vi "Motion_xbee_1Radar.vi"(0 "VISA resource name":refnum<visa-resource-name>="COM1", 1 "baud rate":u32=9600, 4 "data bits":u16=8 min=5 max=8 step=1, 5 "parity":u16(ring) items=["None", "Odd", "Even", "Mark", "Space"], 7 "stop bits":u16=10, 9 "XON Character":u8=17 format="%.0x", 14 "XOFF Character":u8=19 format="%.0x", 15 "timeout (ms)":u32=10000, 21 "End read on termination character?":bool, 24 "termination char\n(0xA = '\\n' = LF)":u8=10 format="%.0x", 25 "buffer size":u32=4096) -> ()   [LabVIEW 2015]
doc: "The Advanced Serial Read and Write example performs a Serial Port Read, a Serial Port Write, or a combination of these actions while setting some advanced serial features like buffer size, termination characters, and XON/XOFF flow control. The user selects the actions (read or write) on the front panel. If both are selected, the VI will write the data first, read the data and then close the VISA session that is opened to the port. \n\nThe parameters set for the serial port must match the parameters of the connected instrument or device. In this example, the bytes to read parameter specifies the number of bytes that the serial port reads. If there were more bytes at the port than the number specified in bytes to read, those bytes would not be read. Also, if you specify to read more bytes than the number of bytes actually read, you might receive a timeout error message.\n\nINSTRUCTIONS:\n1) Select the serial resource and configuration parameters (baud rate, data bits, parity, stop bits, flow control).\n2) Termination character can be enabled and set. Also, set the required input buffer size prior to running the example.\n3) Select the operations to be performed. \n4) Connect the serial port to your device. If no device is available, perform a loopback test by doing one of the following. Short pins 2 and 3 on a RS-232 cable or short pin 4 to pin 8 and pin 5 to pin 9 on a RS-485/422 cable. \n5) Run the VI to see the data read. (The \"read string\" will match the \"string to write\" if a loopback test was performed.)\n\nThis example exposes several advanced features that you may need for your application. Not all applications need all the features shown in this example. The input buffer size is likely an important setting that you want to control in your application. This example expands upon the flow control option for XON and XOFF, allowing the user to choose those control characters. The timeout parameter has been brought to the front panel so a user can specify the time period the VISA Read will wait for the number of bytes to read before timing out. Also, the user has several controls for the termination character, which is discussed later.\n\nNote that you can press the write and read buttons and change the bytes to read parameters on the fly, while the example is running. However, you must stop the example to change the other configuration parameters after the example has started running, and then run again.\n\nSet the I/O buffer size slightly higher the amount of data you expect to receive. This is very important for applications that don't use flow control, as you may lose characters if the receive buffer overflows.\n\nSetting the timeout period ensures that the operation returns with a timeout error if the operation cannot be performed in the specified time period. \n\nSome devices require a termination character in order to identify the end of command strings. Some devices send a termination character to signify the end of data to be read. \n\nThis example shows how you can end the Read operation once a termination character is detected in the buffer and/or append a termination character at the end of the Write data. To enable the Read to end on a termination character, use the VISA Configure Serial Port or use the VISA Properties Serial End Mode for Reads, Termination Character Enable, and Termination Character. To end the Write with a termination character, use the VISA Properties Serial End Mode for Writes, the Send End Enable, and Termination Character. In this example, the same termination character is used for both the Read and the Write. You can specify two different characters for your application, if desired.\n\nYour application may require specific characters for the XON/XOFF Flow Control. You can specify these characters with the VISA Properties Flow Control XOFF Character and Flow Control XON Character. Note that if the standard XON and XOFF characters are used, then decimal 17 and 19 are unavailable for data values. Remember that using flow control and setting an adequate buffer size allow you to prevent buffer overflows."
uses:
  <vilib>/Analysis/2dsp.llb/Real FFT.vi
  <vilib>/Instr/_visa.llb/VISA Configure Serial Port (Instr).vi
  <vilib>/measure/madcrms.llb/Basic Averaged DC-RMS for 1 Chan.vi
  <vilib>/measure/NI_MAPro.lvlib
  <vilib>/Analysis/NI_AALPro.lvlib
panel:
  in  "Data saving path":path=path "C:/Users/zpeng/OneDrive - Texas Tech University/Desktop"
  in  "Save raw data":bool
  out "Spectrum":waveform(dbl)(graph)
  out "I/Q channels":waveform(dbl)(graph)
  in  "time":timestamp=timestamp(3198752888.296 s since 1904-01-01)
  in  "FFT":i32=800
  in  "flow control":u16(ring) items=["None"=0, "XON/XOFF"=1, "RTS/CTS"=2, "DTR/DSR"=4]
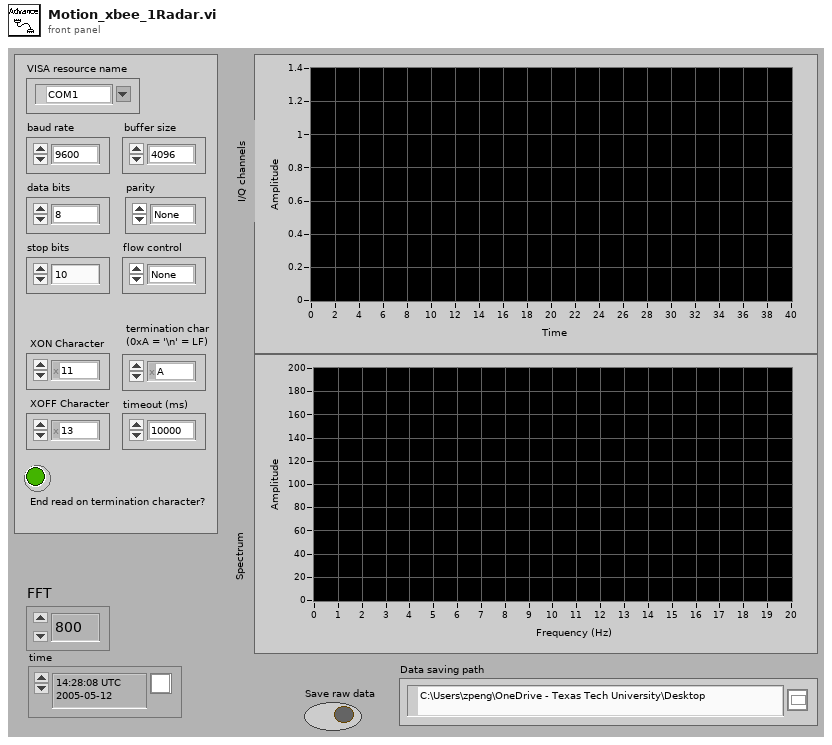
[diagram p1: front panel]
types:
  T1 = enum16{"open", "replace", "create", "open or create", "replace or create", "replace or create with confirmation"}
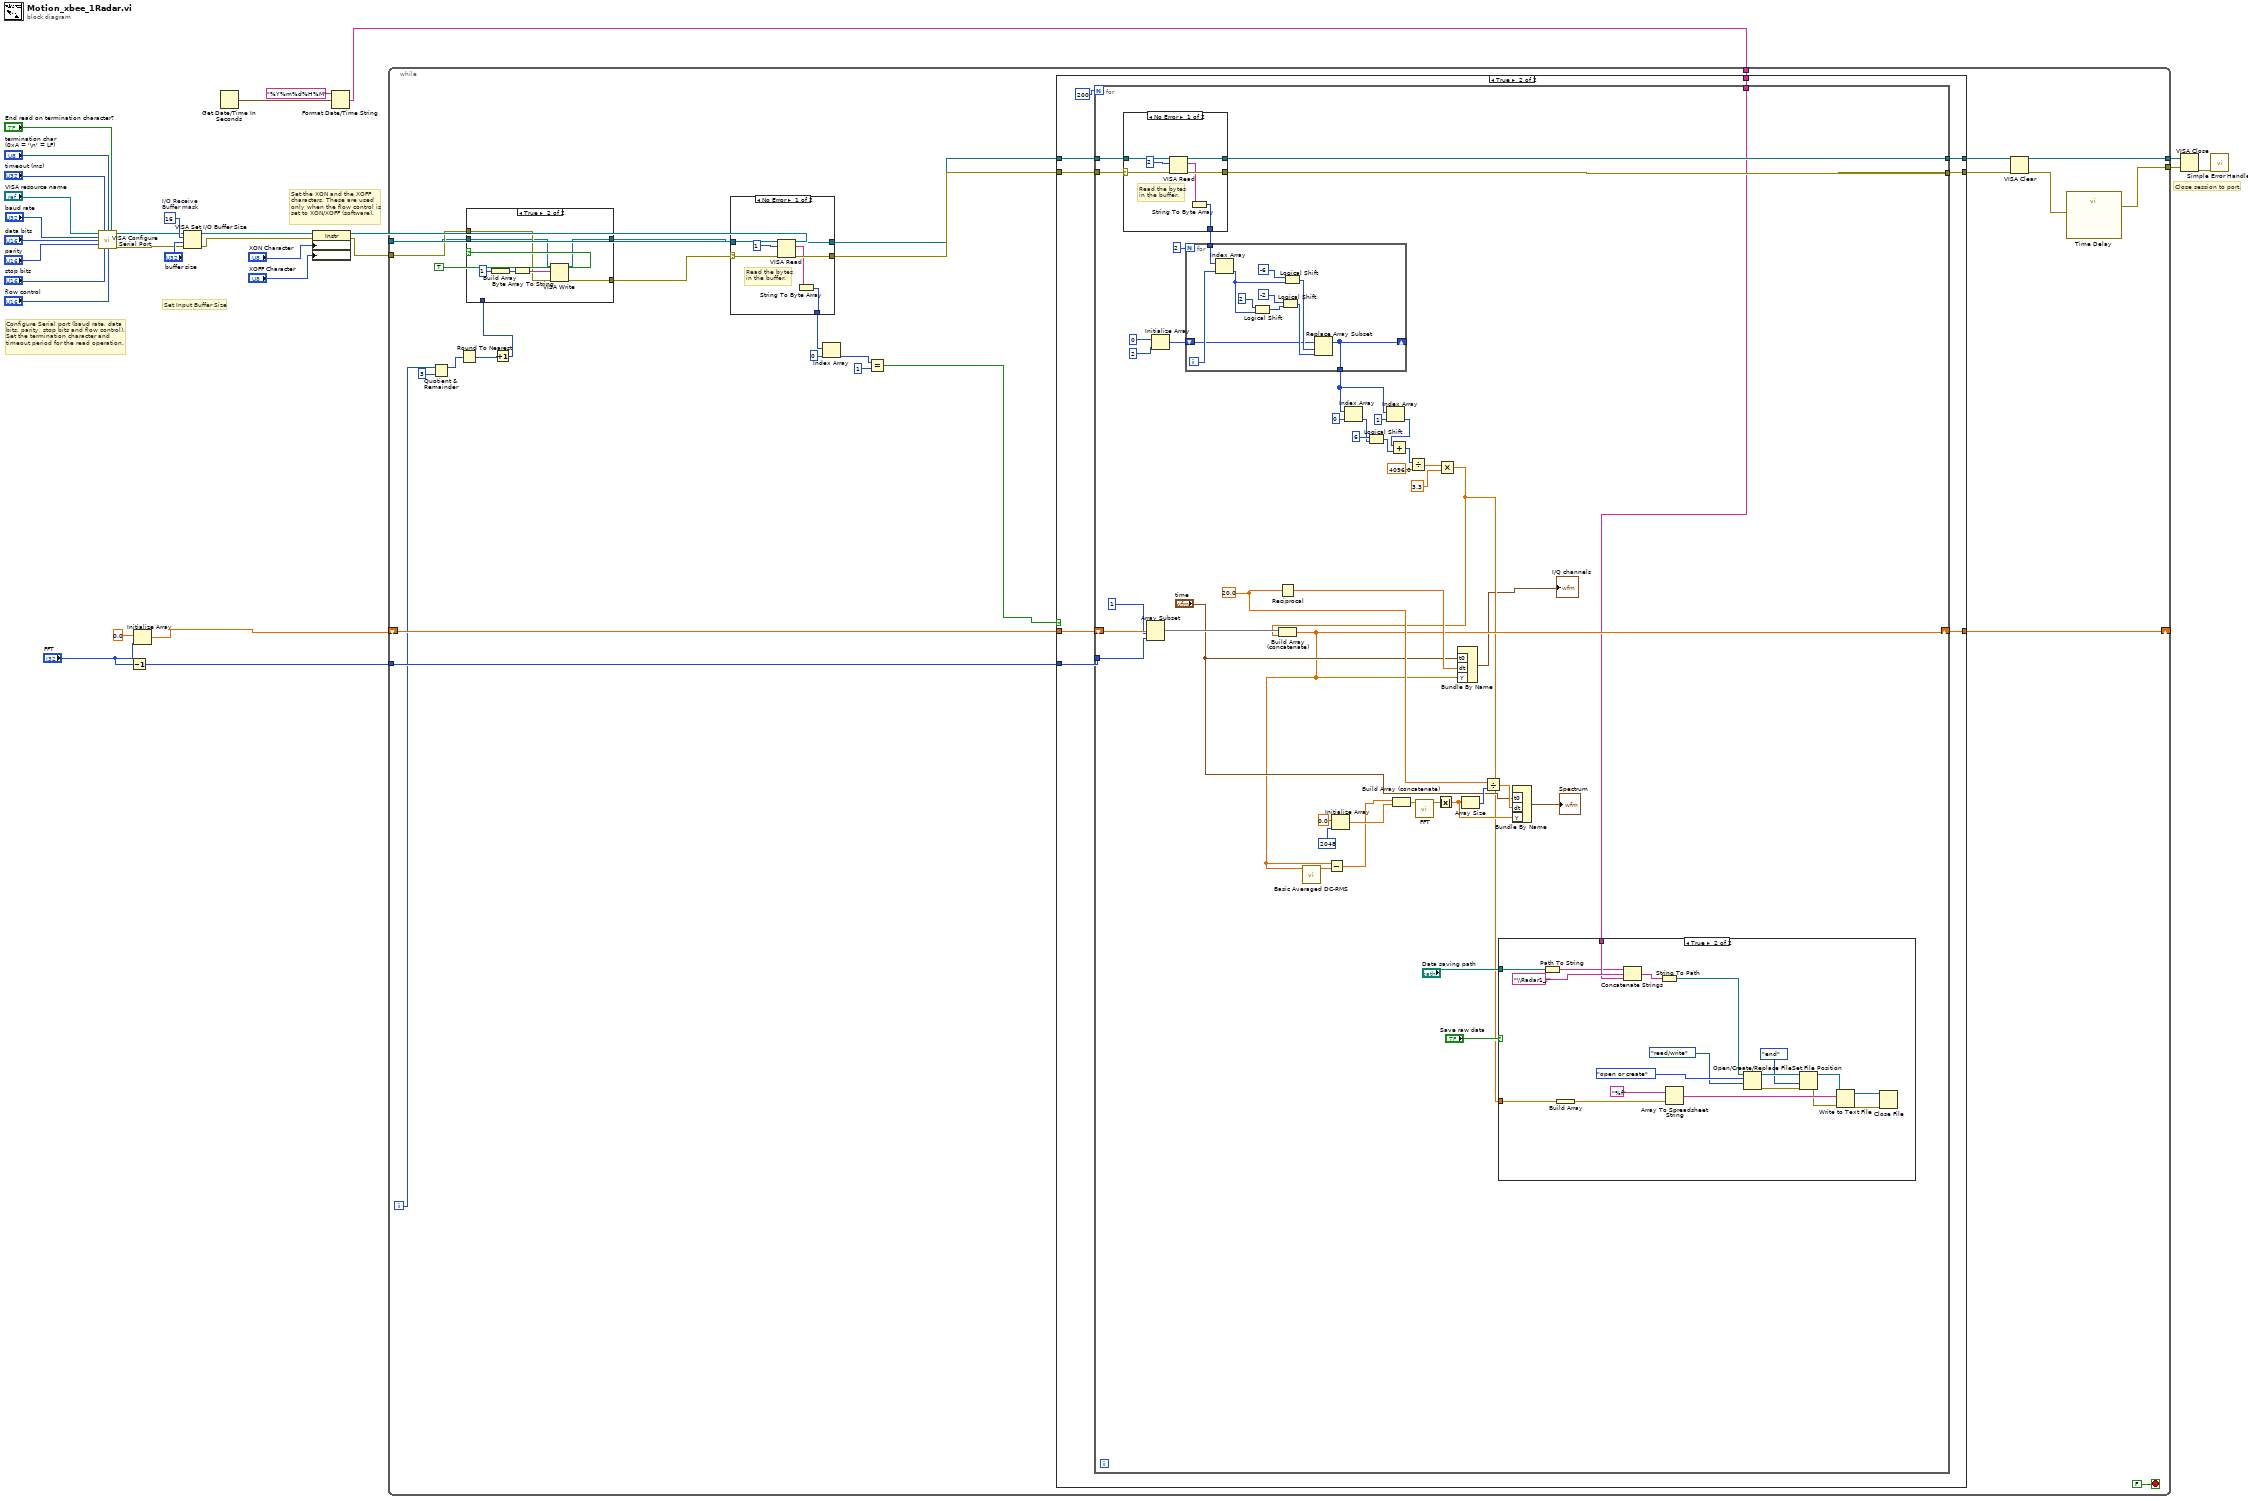
[diagram p0: block diagram]
diagram:
  w22 = u16 16  # I/O Receive Buffer mask
  # "Set the XON and the XOFF\ncharacters. These are used\nonly when the flow control is\nset to XON/XOFF (software)."
  # "Configure Serial port (baud rate, data\nbits, parity, stop bits and flow control).\nSet the termination character and\ntimeout period for the read operation."
  # "Set Input Buffer Size"
  # "Close session to port."
  n1 = call-poly "VISA Configure Serial Port"("VISA resource name"="VISA resource name", "timeout (10sec)"="timeout (ms)", "termination char\n(0xA = '\\n' = LF)"="termination char\n(0xA = '\\n' = LF)", "Enable Termination\nChar (T)"="End read on termination character?", "baud rate (9600)"="baud rate", "data bits (8)"="data bits", "parity (0:none)"="parity", "stop bits (10: 1 bit)"="stop bits", "flow control (0:none)"="flow control") -> ("VISA resource name out"=w8:refnum<visa-resource-name>, "error out"=w7:errorcluster)  [unwired: 1 in, 4 out]
  n2 = Decrement(x="FFT") -> (x-1=w11:i32)
  n3 = Initialize Array(0.0 ("element"), "FFT") -> (w6:dbl[])
  n4 = VISA Set I/O Buffer Size(VISA resource name=w8, mask (16)=w22, size (4096)="buffer size", error in (no error)=w7) -> (VISA resource name out=w18:refnum<visa-resource-name>, error out=w17:errorcluster)
  n5 = Get Date/Time In Seconds() -> (seconds since 1Jan1904=w2:timestamp)
  n6 = property class="Instr"(reference=w18, error in=w17, "Serial Settings:Flow Control XON Character"="XON Character", "Serial Settings:Flow Control XOFF Character"="XOFF Character") -> (reference out=w5:refnum<visa-resource-name>, error out=w4:errorcluster)
  n7 = Format Date/Time String(time format string (%c)="%Y%m%d%H%M", seconds (now)=w2) -> (date/time string=w1:string)  [unwired: 1 in]
  n8 = while {
    tunnel: w11 -> [w56]
    tunnel: w5 -> [w51]
    tunnel: [w45] -> w13
    tunnel: w4 -> [w52]
    tunnel: [w49] -> w12
    shift-right: [w53] -> _
    shift-left: w6 -> [w55]
    tunnel: w1 -> [w30]
    i -> [w34]
    stop <- FALSE stop-if-true
    n9 = Quotient & Remainder(x=w34, y=3) -> (x-y*floor(x/y)=w35:i32)  [unwired: 1 out]
    n10 = Round To Nearest(number=w35) -> (nearest integer value=w32:i32)
    n11 = Increment(x=w32) -> (x+1=w31:i32)
    n12 = case shown="True" TRUE {
      tunnel: w52 -> [w164 w170]
      tunnel: w51 -> [w163 w169]
      tunnel: [w163 w168] -> w43
      tunnel: [w164 w167] -> w44
      tunnel: w31 -> [_ _]
      frame False {
      }
      frame True {
        n13 = Build Array(u8 1 ("element")) -> (w166:u8[])
        n14 = Byte Array To String(unsigned byte array=w166) -> (string=w171:string)
        n15 = VISA Write(VISA resource name=w169, write buffer=w171, error in (no error)=w170) -> (VISA resource name out=w168:refnum<visa-resource-name>, error out=w167:errorcluster)  [unwired: 1 out]
      }
    }
    n16 = case "Read bytes from port." shown="No Error" w44 {
      selector: w44 -> [w60 w65]
      tunnel: [w62 w65] -> w42
      tunnel: [w63 w66] -> w41
      tunnel: w43 -> [w61 w66]
      tunnel: [w58 u8[] [] ("unsigned byte array")] -> w40
      frame No Error {
        # "Read the bytes\nin the buffer."
        n17 = VISA Read(VISA resource name=w61, byte count=u32 1, error in (no error)=w60) -> (VISA resource name out=w63:refnum<visa-resource-name>, read buffer=w59:string, error out=w62:errorcluster)  [unwired: 1 out]
        n18 = String To Byte Array(string=w59) -> (unsigned byte array=w58:u8[])
      }
      frame Error {
        # "Error occurred \nreading Bytes at \nSerial Port"
      }
    }
    n19 = Index Array(array=w40, index=0) -> (element=w38:u8)
    n20 = Equal?(x=w38, y=u8 1) -> (x = y?=w36:bool)
    n21 = case shown="True" w36 {
      tunnel: w56 -> [_ w78]
      tunnel: w55 -> [w67 w76]
      tunnel: [w67 w75] -> w53
      tunnel: [w69 w74] -> w48
      tunnel: w41 -> [w69 w73]
      tunnel: w42 -> [w68 w72]
      tunnel: [w68 w71] -> w47
      tunnel: w30 -> [_ w70]
      frame False {
      }
      frame True {
        n22 = for {
          N: 200 -> [_]
          tunnel: w72 -> [w108]
          tunnel: w73 -> [w107]
          tunnel: [w87] -> w74
          tunnel: [w86] -> w71
          tunnel: w78 -> [w114]
          shift-right: [w92] -> w75
          shift-left: w76 -> [w121]
          tunnel: w70 -> [w82]
          (unwired) 0
          w100 = 20.0 ("dt")
          n23 = case "Read bytes from port." shown="No Error" w108 {
            selector: w108 -> [w156 w161]
            tunnel: [w158 w161] -> w86
            tunnel: [w159 w162] -> w87
            tunnel: w107 -> [w157 w162]
            tunnel: [w154 u8[] [] ("unsigned byte array")] -> w88
            frame No Error {
              # "Read the bytes\nin the buffer."
              n24 = VISA Read(VISA resource name=w157, byte count=u32 2, error in (no error)=w156) -> (VISA resource name out=w159:refnum<visa-resource-name>, read buffer=w155:string, error out=w158:errorcluster)  [unwired: 1 out]
              n25 = String To Byte Array(string=w155) -> (unsigned byte array=w154:u8[])
            }
            frame Error {
              # "Error occurred \nreading Bytes at \nSerial Port"
            }
          }
          n26 = Array Subset(array=w121, index=1, length=w114) -> (w122:dbl[])
          n27 = Initialize Array(i16 0 ("element"), 2 ("dimension size")) -> (w89:i16[])
          n28 = for {
            N: 2 -> [_]
            tunnel: w88 -> [w147]
            tunnel: [w142] -> w94
            shift-right: [w142] -> _
            shift-left: w89 -> [w143]
            i -> [w146]
            n29 = Index Array(array=w147, index=w146) -> (element=w150:u8)
            n30 = Logical Shift(y=i8 2, x=w150) -> (x << y=w149:u8)
            n31 = Logical Shift(y=i8 -2, x=w149) -> (x << y=w144:u8)
            n32 = Logical Shift(y=i8 -6, x=w150) -> (x << y=w145:u8)
            n33 = Replace Array Subset(array=w143, new element=w144, index=w145) -> (w142:i16[])
          }
          n34 = Reciprocal(x=w100) -> (1/x=w109:dbl)
          n35 = Initialize Array(0.0 ("element"), 2048 ("dimension size")) -> (w103:dbl[])
          n36 = Index Array(array=w94, index=0) -> (element=w117:i16)
          n37 = Logical Shift(y=i16 6, x=w117) -> (x << y=w115:i16)
          n38 = Index Array(array=w94, index=1) -> (element=w116:i16)
          n39 = Add(x=w116, y=w115) -> (x+y=w85:i16)
          n40 = Divide(x=w85, y=4096.0) -> (x/y=w112:dbl)
          n41 = Multiply(x=w112, y=3.3) -> (x*y=w81:dbl)
          n42 = Build Array (concatenate)(w122, w81) -> (w92:dbl[])
          n43 = call-poly <vilib>:"Basic Averaged DC-RMS.vi"("signal in"=w92) -> ("DC value"=w111:dbl)  [unwired: 4 in, 6 out]
          n44 = Subtract(x=w92, y=w111) -> (x-y=w79:dbl[])
          n45 = Build Array (concatenate)(w79, w103) -> (w104:dbl[])
          n46 = call-poly <vilib>:"FFT.vi"("X"=w104) -> ("FFT {X}"=w101:cdb[])  [unwired: 2 in, 8 out]
          n47 = Absolute Value(x=w101) -> (abs(x)=w99:dbl[])
          n48 = Bundle By Name ("Build Waveform")("t0"="time", "dt"=w109, "Y"=w92) -> (→"I/Q channels":waveform(dbl))  [unwired: 1 out]
          n49 = Array Size(array=w99) -> (size(s)=w102:i32)
          n50 = Divide(x=w100, y=w102) -> (x/y=w98:dbl)
          n51 = case shown="True" "Save raw data" {
            tunnel: w81 -> [_ w135]
            tunnel: w82 -> [_ w137]
            tunnel: "Data saving path" -> [_ w136]
            frame False {
            }
            frame True {
              n52 = Path To String(path=w136) -> (string=w123:string)
              n53 = Build Array(w135) -> (w124:dbl[])
              n54 = Concatenate Strings(w123, "\\Radar1_I" ("string"), w137) -> (w141:string)
              n55 = String To Path(string=w141) -> (path=w134:path)
              n56 = Array To Spreadsheet String(array=w124, 3:"%f" ("format string")) -> (spreadsheet string=w140:string)  [unwired: 1 in]
              n57 = Open/Create/Replace File(file path (use dialog)=w134, operation (0:open)=T1."open or create", access (0:read/write)=enum16{"read/write", "read-only", "write-only"}."read/write") -> (refnum out=w133:refnum<file>, error out=w132:errorcluster)  [unwired: 3 in, 1 out]
              n58 = Set File Position(refnum=w133, from (0:start)=enum16{"start", "end", "current"}."end", error in=w132) -> (refnum out=w131:refnum<file>, error out=w130:errorcluster)  [unwired: 1 in]
              n59 = Write to Text File(file (use dialog)=w131, text=w140, error in=w130) -> (refnum out=w128:refnum<file>, error out=w127:errorcluster)  [unwired: 1 in, 1 out]
              n60 = Close File(refnum=w128, error in=w127) -> ()  [unwired: 2 out]
            }
          }
          n61 = Bundle By Name("t0"="time", "dt"=w98, "Y"=w99) -> (→"Spectrum":waveform(dbl))  [unwired: 1 out]
        }
      }
    }
    n62 = VISA Clear(VISA resource name=w48, error in (no error)=w47) -> (VISA resource name out=w45:refnum<visa-resource-name>, error out=w46:errorcluster)
    n63 = call "Time Delay"("error in (no error)"=w46) -> ("error out"=w49:errorcluster)  [unwired: 10 in]
  }
  n64 = VISA Close(VISA resource name=w13, error in (no error)=w12) -> (error out=w27:errorcluster)
  n65 = call <vilib>:"Simple Error Handler.vi"("error in (no error)"=w27) -> ()  [unwired: 1 in, 8 out]
